vi "Main.vi"() -> ()   [LabVIEW 2021] (continued)
                    w2240 = T9 81 items=["刷新间隔", "波特率", "布尔1设置项", "布尔2设置项", "布尔3设置项", "布尔4设置项", "布尔5设置项", "布尔6设置项", "布尔7设置项", "布尔8设置项", "显控1设置", "显控2设置", "显控3设置", "显控4设置", "显控5设置", "显控6设置", "显控7设置", "显控8设置", "显控9设置", "显控10设置", "显控11设置", "显控12设置", "设控1设置", "设控2设置", "设控3设置", "设控4设置", "设控5设置", "设控6设置", "设控7设置", "设控8设置", "曲线1设置", "曲线2设置", "曲线3设置", "曲线4设置", "曲线5设置", "曲线6设置", "曲线7设置", "曲线8设置", "曲线9设置", "曲线10设置", "曲线11设置", "曲线12设置", "曲线13设置", "曲线14设置", "曲线15设置", "曲线16设置", "曲线17设置", "曲线18设置", "曲线19设置", "曲线20设置", "曲线21设置", "曲线22设置", "曲线23设置", "曲线24设置", "曲线25设置", "曲线26设置", "曲线27设置", "曲线28设置", "曲线29设置", "曲线30设置", "曲线31设置", "曲线32设置", "曲线33设置", "曲线34设置", "曲线35设置", "曲线36设置", "曲线37设置", "曲线38设置", "曲线39设置", "曲线40设置", "曲线41设置", "曲线42设置", "曲线43设置", "曲线44设置", "曲线45设置", "曲线46设置", "曲线47设置", "曲线48设置", "曲线49设置", "曲线50设置", "曲线51设置", "曲线52设置", "曲线53设置", "曲线54设置", "曲线55设置", "曲线56设置", "曲线57设置", "曲线58设置", "曲线59设置", "曲线60设置", "曲线61设置", "曲线62设置", "曲线63设置", "曲线64设置", "ID值", "数据模式"] ("DataInitDef")
                    w2244 = "曲线52" ("值")
                    n1732 = invoke on="控件配置文件" class="Tbl (严格)" method="Set Cell Value"("X Index"=1 ("X索引"), "Y Index"=w2240, "Value"="X" ("值")) -> ()  [unwired: 3 in, 6 out]
                    n1733 = invoke on="控件配置文件" class="Tbl (严格)" method="Set Cell Value"("X Index"=0 ("X索引"), "Y Index"=w2240, "Value"=w2244) -> ()  [unwired: 3 in, 6 out]
                    n1734 = property on="曲线52设置" class="Str"("Val(Sgnl)"=w2244) -> ()  [unwired: 2 in, 2 out]
                  }
                  frame "删除曲线53" {
                    w2245 = T9 82 items=["刷新间隔", "波特率", "布尔1设置项", "布尔2设置项", "布尔3设置项", "布尔4设置项", "布尔5设置项", "布尔6设置项", "布尔7设置项", "布尔8设置项", "显控1设置", "显控2设置", "显控3设置", "显控4设置", "显控5设置", "显控6设置", "显控7设置", "显控8设置", "显控9设置", "显控10设置", "显控11设置", "显控12设置", "设控1设置", "设控2设置", "设控3设置", "设控4设置", "设控5设置", "设控6设置", "设控7设置", "设控8设置", "曲线1设置", "曲线2设置", "曲线3设置", "曲线4设置", "曲线5设置", "曲线6设置", "曲线7设置", "曲线8设置", "曲线9设置", "曲线10设置", "曲线11设置", "曲线12设置", "曲线13设置", "曲线14设置", "曲线15设置", "曲线16设置", "曲线17设置", "曲线18设置", "曲线19设置", "曲线20设置", "曲线21设置", "曲线22设置", "曲线23设置", "曲线24设置", "曲线25设置", "曲线26设置", "曲线27设置", "曲线28设置", "曲线29设置", "曲线30设置", "曲线31设置", "曲线32设置", "曲线33设置", "曲线34设置", "曲线35设置", "曲线36设置", "曲线37设置", "曲线38设置", "曲线39设置", "曲线40设置", "曲线41设置", "曲线42设置", "曲线43设置", "曲线44设置", "曲线45设置", "曲线46设置", "曲线47设置", "曲线48设置", "曲线49设置", "曲线50设置", "曲线51设置", "曲线52设置", "曲线53设置", "曲线54设置", "曲线55设置", "曲线56设置", "曲线57设置", "曲线58设置", "曲线59设置", "曲线60设置", "曲线61设置", "曲线62设置", "曲线63设置", "曲线64设置", "ID值", "数据模式"] ("DataInitDef")
                    w2249 = "曲线53" ("值")
                    n1735 = invoke on="控件配置文件" class="Tbl (严格)" method="Set Cell Value"("X Index"=1 ("X索引"), "Y Index"=w2245, "Value"="X" ("值")) -> ()  [unwired: 3 in, 6 out]
                    n1736 = invoke on="控件配置文件" class="Tbl (严格)" method="Set Cell Value"("X Index"=0 ("X索引"), "Y Index"=w2245, "Value"=w2249) -> ()  [unwired: 3 in, 6 out]
                    n1737 = property on="曲线53设置" class="Str"("Val(Sgnl)"=w2249) -> ()  [unwired: 2 in, 2 out]
                  }
                  frame "删除曲线54" {
                    w2250 = T9 83 items=["刷新间隔", "波特率", "布尔1设置项", "布尔2设置项", "布尔3设置项", "布尔4设置项", "布尔5设置项", "布尔6设置项", "布尔7设置项", "布尔8设置项", "显控1设置", "显控2设置", "显控3设置", "显控4设置", "显控5设置", "显控6设置", "显控7设置", "显控8设置", "显控9设置", "显控10设置", "显控11设置", "显控12设置", "设控1设置", "设控2设置", "设控3设置", "设控4设置", "设控5设置", "设控6设置", "设控7设置", "设控8设置", "曲线1设置", "曲线2设置", "曲线3设置", "曲线4设置", "曲线5设置", "曲线6设置", "曲线7设置", "曲线8设置", "曲线9设置", "曲线10设置", "曲线11设置", "曲线12设置", "曲线13设置", "曲线14设置", "曲线15设置", "曲线16设置", "曲线17设置", "曲线18设置", "曲线19设置", "曲线20设置", "曲线21设置", "曲线22设置", "曲线23设置", "曲线24设置", "曲线25设置", "曲线26设置", "曲线27设置", "曲线28设置", "曲线29设置", "曲线30设置", "曲线31设置", "曲线32设置", "曲线33设置", "曲线34设置", "曲线35设置", "曲线36设置", "曲线37设置", "曲线38设置", "曲线39设置", "曲线40设置", "曲线41设置", "曲线42设置", "曲线43设置", "曲线44设置", "曲线45设置", "曲线46设置", "曲线47设置", "曲线48设置", "曲线49设置", "曲线50设置", "曲线51设置", "曲线52设置", "曲线53设置", "曲线54设置", "曲线55设置", "曲线56设置", "曲线57设置", "曲线58设置", "曲线59设置", "曲线60设置", "曲线61设置", "曲线62设置", "曲线63设置", "曲线64设置", "ID值", "数据模式"] ("DataInitDef")
                    w2254 = "曲线54" ("值")
                    n1738 = invoke on="控件配置文件" class="Tbl (严格)" method="Set Cell Value"("X Index"=1 ("X索引"), "Y Index"=w2250, "Value"="X" ("值")) -> ()  [unwired: 3 in, 6 out]
                    n1739 = invoke on="控件配置文件" class="Tbl (严格)" method="Set Cell Value"("X Index"=0 ("X索引"), "Y Index"=w2250, "Value"=w2254) -> ()  [unwired: 3 in, 6 out]
                    n1740 = property on="曲线54设置" class="Str"("Val(Sgnl)"=w2254) -> ()  [unwired: 2 in, 2 out]
                  }
                  frame "删除曲线55" {
                    w2255 = T9 84 items=["刷新间隔", "波特率", "布尔1设置项", "布尔2设置项", "布尔3设置项", "布尔4设置项", "布尔5设置项", "布尔6设置项", "布尔7设置项", "布尔8设置项", "显控1设置", "显控2设置", "显控3设置", "显控4设置", "显控5设置", "显控6设置", "显控7设置", "显控8设置", "显控9设置", "显控10设置", "显控11设置", "显控12设置", "设控1设置", "设控2设置", "设控3设置", "设控4设置", "设控5设置", "设控6设置", "设控7设置", "设控8设置", "曲线1设置", "曲线2设置", "曲线3设置", "曲线4设置", "曲线5设置", "曲线6设置", "曲线7设置", "曲线8设置", "曲线9设置", "曲线10设置", "曲线11设置", "曲线12设置", "曲线13设置", "曲线14设置", "曲线15设置", "曲线16设置", "曲线17设置", "曲线18设置", "曲线19设置", "曲线20设置", "曲线21设置", "曲线22设置", "曲线23设置", "曲线24设置", "曲线25设置", "曲线26设置", "曲线27设置", "曲线28设置", "曲线29设置", "曲线30设置", "曲线31设置", "曲线32设置", "曲线33设置", "曲线34设置", "曲线35设置", "曲线36设置", "曲线37设置", "曲线38设置", "曲线39设置", "曲线40设置", "曲线41设置", "曲线42设置", "曲线43设置", "曲线44设置", "曲线45设置", "曲线46设置", "曲线47设置", "曲线48设置", "曲线49设置", "曲线50设置", "曲线51设置", "曲线52设置", "曲线53设置", "曲线54设置", "曲线55设置", "曲线56设置", "曲线57设置", "曲线58设置", "曲线59设置", "曲线60设置", "曲线61设置", "曲线62设置", "曲线63设置", "曲线64设置", "ID值", "数据模式"] ("DataInitDef")
                    w2259 = "曲线55" ("值")
                    n1741 = invoke on="控件配置文件" class="Tbl (严格)" method="Set Cell Value"("X Index"=1 ("X索引"), "Y Index"=w2255, "Value"="X" ("值")) -> ()  [unwired: 3 in, 6 out]
                    n1742 = invoke on="控件配置文件" class="Tbl (严格)" method="Set Cell Value"("X Index"=0 ("X索引"), "Y Index"=w2255, "Value"=w2259) -> ()  [unwired: 3 in, 6 out]
                    n1743 = property on="曲线55设置" class="Str"("Val(Sgnl)"=w2259) -> ()  [unwired: 2 in, 2 out]
                  }
                  frame "删除曲线56" {
                    w2260 = T9 85 items=["刷新间隔", "波特率", "布尔1设置项", "布尔2设置项", "布尔3设置项", "布尔4设置项", "布尔5设置项", "布尔6设置项", "布尔7设置项", "布尔8设置项", "显控1设置", "显控2设置", "显控3设置", "显控4设置", "显控5设置", "显控6设置", "显控7设置", "显控8设置", "显控9设置", "显控10设置", "显控11设置", "显控12设置", "设控1设置", "设控2设置", "设控3设置", "设控4设置", "设控5设置", "设控6设置", "设控7设置", "设控8设置", "曲线1设置", "曲线2设置", "曲线3设置", "曲线4设置", "曲线5设置", "曲线6设置", "曲线7设置", "曲线8设置", "曲线9设置", "曲线10设置", "曲线11设置", "曲线12设置", "曲线13设置", "曲线14设置", "曲线15设置", "曲线16设置", "曲线17设置", "曲线18设置", "曲线19设置", "曲线20设置", "曲线21设置", "曲线22设置", "曲线23设置", "曲线24设置", "曲线25设置", "曲线26设置", "曲线27设置", "曲线28设置", "曲线29设置", "曲线30设置", "曲线31设置", "曲线32设置", "曲线33设置", "曲线34设置", "曲线35设置", "曲线36设置", "曲线37设置", "曲线38设置", "曲线39设置", "曲线40设置", "曲线41设置", "曲线42设置", "曲线43设置", "曲线44设置", "曲线45设置", "曲线46设置", "曲线47设置", "曲线48设置", "曲线49设置", "曲线50设置", "曲线51设置", "曲线52设置", "曲线53设置", "曲线54设置", "曲线55设置", "曲线56设置", "曲线57设置", "曲线58设置", "曲线59设置", "曲线60设置", "曲线61设置", "曲线62设置", "曲线63设置", "曲线64设置", "ID值", "数据模式"] ("DataInitDef")
                    w2264 = "曲线56" ("值")
                    n1744 = invoke on="控件配置文件" class="Tbl (严格)" method="Set Cell Value"("X Index"=1 ("X索引"), "Y Index"=w2260, "Value"="X" ("值")) -> ()  [unwired: 3 in, 6 out]
                    n1745 = invoke on="控件配置文件" class="Tbl (严格)" method="Set Cell Value"("X Index"=0 ("X索引"), "Y Index"=w2260, "Value"=w2264) -> ()  [unwired: 3 in, 6 out]
                    n1746 = property on="曲线56设置" class="Str"("Val(Sgnl)"=w2264) -> ()  [unwired: 2 in, 2 out]
                  }
                  frame "删除曲线57" {
                    w2265 = T9 86 items=["刷新间隔", "波特率", "布尔1设置项", "布尔2设置项", "布尔3设置项", "布尔4设置项", "布尔5设置项", "布尔6设置项", "布尔7设置项", "布尔8设置项", "显控1设置", "显控2设置", "显控3设置", "显控4设置", "显控5设置", "显控6设置", "显控7设置", "显控8设置", "显控9设置", "显控10设置", "显控11设置", "显控12设置", "设控1设置", "设控2设置", "设控3设置", "设控4设置", "设控5设置", "设控6设置", "设控7设置", "设控8设置", "曲线1设置", "曲线2设置", "曲线3设置", "曲线4设置", "曲线5设置", "曲线6设置", "曲线7设置", "曲线8设置", "曲线9设置", "曲线10设置", "曲线11设置", "曲线12设置", "曲线13设置", "曲线14设置", "曲线15设置", "曲线16设置", "曲线17设置", "曲线18设置", "曲线19设置", "曲线20设置", "曲线21设置", "曲线22设置", "曲线23设置", "曲线24设置", "曲线25设置", "曲线26设置", "曲线27设置", "曲线28设置", "曲线29设置", "曲线30设置", "曲线31设置", "曲线32设置", "曲线33设置", "曲线34设置", "曲线35设置", "曲线36设置", "曲线37设置", "曲线38设置", "曲线39设置", "曲线40设置", "曲线41设置", "曲线42设置", "曲线43设置", "曲线44设置", "曲线45设置", "曲线46设置", "曲线47设置", "曲线48设置", "曲线49设置", "曲线50设置", "曲线51设置", "曲线52设置", "曲线53设置", "曲线54设置", "曲线55设置", "曲线56设置", "曲线57设置", "曲线58设置", "曲线59设置", "曲线60设置", "曲线61设置", "曲线62设置", "曲线63设置", "曲线64设置", "ID值", "数据模式"] ("DataInitDef")
                    w2269 = "曲线57" ("值")
                    n1747 = invoke on="控件配置文件" class="Tbl (严格)" method="Set Cell Value"("X Index"=1 ("X索引"), "Y Index"=w2265, "Value"="X" ("值")) -> ()  [unwired: 3 in, 6 out]
                    n1748 = invoke on="控件配置文件" class="Tbl (严格)" method="Set Cell Value"("X Index"=0 ("X索引"), "Y Index"=w2265, "Value"=w2269) -> ()  [unwired: 3 in, 6 out]
                    n1749 = property on="曲线57设置" class="Str"("Val(Sgnl)"=w2269) -> ()  [unwired: 2 in, 2 out]
                  }
                  frame "删除曲线58" {
                    w2270 = T9 87 items=["刷新间隔", "波特率", "布尔1设置项", "布尔2设置项", "布尔3设置项", "布尔4设置项", "布尔5设置项", "布尔6设置项", "布尔7设置项", "布尔8设置项", "显控1设置", "显控2设置", "显控3设置", "显控4设置", "显控5设置", "显控6设置", "显控7设置", "显控8设置", "显控9设置", "显控10设置", "显控11设置", "显控12设置", "设控1设置", "设控2设置", "设控3设置", "设控4设置", "设控5设置", "设控6设置", "设控7设置", "设控8设置", "曲线1设置", "曲线2设置", "曲线3设置", "曲线4设置", "曲线5设置", "曲线6设置", "曲线7设置", "曲线8设置", "曲线9设置", "曲线10设置", "曲线11设置", "曲线12设置", "曲线13设置", "曲线14设置", "曲线15设置", "曲线16设置", "曲线17设置", "曲线18设置", "曲线19设置", "曲线20设置", "曲线21设置", "曲线22设置", "曲线23设置", "曲线24设置", "曲线25设置", "曲线26设置", "曲线27设置", "曲线28设置", "曲线29设置", "曲线30设置", "曲线31设置", "曲线32设置", "曲线33设置", "曲线34设置", "曲线35设置", "曲线36设置", "曲线37设置", "曲线38设置", "曲线39设置", "曲线40设置", "曲线41设置", "曲线42设置", "曲线43设置", "曲线44设置", "曲线45设置", "曲线46设置", "曲线47设置", "曲线48设置", "曲线49设置", "曲线50设置", "曲线51设置", "曲线52设置", "曲线53设置", "曲线54设置", "曲线55设置", "曲线56设置", "曲线57设置", "曲线58设置", "曲线59设置", "曲线60设置", "曲线61设置", "曲线62设置", "曲线63设置", "曲线64设置", "ID值", "数据模式"] ("DataInitDef")
                    w2274 = "曲线58" ("值")
                    n1750 = invoke on="控件配置文件" class="Tbl (严格)" method="Set Cell Value"("X Index"=1 ("X索引"), "Y Index"=w2270, "Value"="X" ("值")) -> ()  [unwired: 3 in, 6 out]
                    n1751 = invoke on="控件配置文件" class="Tbl (严格)" method="Set Cell Value"("X Index"=0 ("X索引"), "Y Index"=w2270, "Value"=w2274) -> ()  [unwired: 3 in, 6 out]
                    n1752 = property on="曲线58设置" class="Str"("Val(Sgnl)"=w2274) -> ()  [unwired: 2 in, 2 out]
                  }
                  frame "删除曲线59" {
                    w2275 = T9 88 items=["刷新间隔", "波特率", "布尔1设置项", "布尔2设置项", "布尔3设置项", "布尔4设置项", "布尔5设置项", "布尔6设置项", "布尔7设置项", "布尔8设置项", "显控1设置", "显控2设置", "显控3设置", "显控4设置", "显控5设置", "显控6设置", "显控7设置", "显控8设置", "显控9设置", "显控10设置", "显控11设置", "显控12设置", "设控1设置", "设控2设置", "设控3设置", "设控4设置", "设控5设置", "设控6设置", "设控7设置", "设控8设置", "曲线1设置", "曲线2设置", "曲线3设置", "曲线4设置", "曲线5设置", "曲线6设置", "曲线7设置", "曲线8设置", "曲线9设置", "曲线10设置", "曲线11设置", "曲线12设置", "曲线13设置", "曲线14设置", "曲线15设置", "曲线16设置", "曲线17设置", "曲线18设置", "曲线19设置", "曲线20设置", "曲线21设置", "曲线22设置", "曲线23设置", "曲线24设置", "曲线25设置", "曲线26设置", "曲线27设置", "曲线28设置", "曲线29设置", "曲线30设置", "曲线31设置", "曲线32设置", "曲线33设置", "曲线34设置", "曲线35设置", "曲线36设置", "曲线37设置", "曲线38设置", "曲线39设置", "曲线40设置", "曲线41设置", "曲线42设置", "曲线43设置", "曲线44设置", "曲线45设置", "曲线46设置", "曲线47设置", "曲线48设置", "曲线49设置", "曲线50设置", "曲线51设置", "曲线52设置", "曲线53设置", "曲线54设置", "曲线55设置", "曲线56设置", "曲线57设置", "曲线58设置", "曲线59设置", "曲线60设置", "曲线61设置", "曲线62设置", "曲线63设置", "曲线64设置", "ID值", "数据模式"] ("DataInitDef")
                    w2279 = "曲线59" ("值")
                    n1753 = invoke on="控件配置文件" class="Tbl (严格)" method="Set Cell Value"("X Index"=1 ("X索引"), "Y Index"=w2275, "Value"="X" ("值")) -> ()  [unwired: 3 in, 6 out]
                    n1754 = invoke on="控件配置文件" class="Tbl (严格)" method="Set Cell Value"("X Index"=0 ("X索引"), "Y Index"=w2275, "Value"=w2279) -> ()  [unwired: 3 in, 6 out]
                    n1755 = property on="曲线59设置" class="Str"("Val(Sgnl)"=w2279) -> ()  [unwired: 2 in, 2 out]
                  }
                  frame "删除曲线60" {
                    w2280 = T9 89 items=["刷新间隔", "波特率", "布尔1设置项", "布尔2设置项", "布尔3设置项", "布尔4设置项", "布尔5设置项", "布尔6设置项", "布尔7设置项", "布尔8设置项", "显控1设置", "显控2设置", "显控3设置", "显控4设置", "显控5设置", "显控6设置", "显控7设置", "显控8设置", "显控9设置", "显控10设置", "显控11设置", "显控12设置", "设控1设置", "设控2设置", "设控3设置", "设控4设置", "设控5设置", "设控6设置", "设控7设置", "设控8设置", "曲线1设置", "曲线2设置", "曲线3设置", "曲线4设置", "曲线5设置", "曲线6设置", "曲线7设置", "曲线8设置", "曲线9设置", "曲线10设置", "曲线11设置", "曲线12设置", "曲线13设置", "曲线14设置", "曲线15设置", "曲线16设置", "曲线17设置", "曲线18设置", "曲线19设置", "曲线20设置", "曲线21设置", "曲线22设置", "曲线23设置", "曲线24设置", "曲线25设置", "曲线26设置", "曲线27设置", "曲线28设置", "曲线29设置", "曲线30设置", "曲线31设置", "曲线32设置", "曲线33设置", "曲线34设置", "曲线35设置", "曲线36设置", "曲线37设置", "曲线38设置", "曲线39设置", "曲线40设置", "曲线41设置", "曲线42设置", "曲线43设置", "曲线44设置", "曲线45设置", "曲线46设置", "曲线47设置", "曲线48设置", "曲线49设置", "曲线50设置", "曲线51设置", "曲线52设置", "曲线53设置", "曲线54设置", "曲线55设置", "曲线56设置", "曲线57设置", "曲线58设置", "曲线59设置", "曲线60设置", "曲线61设置", "曲线62设置", "曲线63设置", "曲线64设置", "ID值", "数据模式"] ("DataInitDef")
                    w2284 = "曲线60" ("值")
                    n1756 = invoke on="控件配置文件" class="Tbl (严格)" method="Set Cell Value"("X Index"=1 ("X索引"), "Y Index"=w2280, "Value"="X" ("值")) -> ()  [unwired: 3 in, 6 out]
                    n1757 = invoke on="控件配置文件" class="Tbl (严格)" method="Set Cell Value"("X Index"=0 ("X索引"), "Y Index"=w2280, "Value"=w2284) -> ()  [unwired: 3 in, 6 out]
                    n1758 = property on="曲线60设置" class="Str"("Val(Sgnl)"=w2284) -> ()  [unwired: 2 in, 2 out]
                  }
                  frame "删除曲线61" {
                    w2285 = T9 90 items=["刷新间隔", "波特率", "布尔1设置项", "布尔2设置项", "布尔3设置项", "布尔4设置项", "布尔5设置项", "布尔6设置项", "布尔7设置项", "布尔8设置项", "显控1设置", "显控2设置", "显控3设置", "显控4设置", "显控5设置", "显控6设置", "显控7设置", "显控8设置", "显控9设置", "显控10设置", "显控11设置", "显控12设置", "设控1设置", "设控2设置", "设控3设置", "设控4设置", "设控5设置", "设控6设置", "设控7设置", "设控8设置", "曲线1设置", "曲线2设置", "曲线3设置", "曲线4设置", "曲线5设置", "曲线6设置", "曲线7设置", "曲线8设置", "曲线9设置", "曲线10设置", "曲线11设置", "曲线12设置", "曲线13设置", "曲线14设置", "曲线15设置", "曲线16设置", "曲线17设置", "曲线18设置", "曲线19设置", "曲线20设置", "曲线21设置", "曲线22设置", "曲线23设置", "曲线24设置", "曲线25设置", "曲线26设置", "曲线27设置", "曲线28设置", "曲线29设置", "曲线30设置", "曲线31设置", "曲线32设置", "曲线33设置", "曲线34设置", "曲线35设置", "曲线36设置", "曲线37设置", "曲线38设置", "曲线39设置", "曲线40设置", "曲线41设置", "曲线42设置", "曲线43设置", "曲线44设置", "曲线45设置", "曲线46设置", "曲线47设置", "曲线48设置", "曲线49设置", "曲线50设置", "曲线51设置", "曲线52设置", "曲线53设置", "曲线54设置", "曲线55设置", "曲线56设置", "曲线57设置", "曲线58设置", "曲线59设置", "曲线60设置", "曲线61设置", "曲线62设置", "曲线63设置", "曲线64设置", "ID值", "数据模式"] ("DataInitDef")
                    w2289 = "曲线61" ("值")
                    n1759 = invoke on="控件配置文件" class="Tbl (严格)" method="Set Cell Value"("X Index"=1 ("X索引"), "Y Index"=w2285, "Value"="X" ("值")) -> ()  [unwired: 3 in, 6 out]
                    n1760 = invoke on="控件配置文件" class="Tbl (严格)" method="Set Cell Value"("X Index"=0 ("X索引"), "Y Index"=w2285, "Value"=w2289) -> ()  [unwired: 3 in, 6 out]
                    n1761 = property on="曲线61设置" class="Str"("Val(Sgnl)"=w2289) -> ()  [unwired: 2 in, 2 out]
                  }
                  frame "删除曲线62" {
                    w2290 = T9 91 items=["刷新间隔", "波特率", "布尔1设置项", "布尔2设置项", "布尔3设置项", "布尔4设置项", "布尔5设置项", "布尔6设置项", "布尔7设置项", "布尔8设置项", "显控1设置", "显控2设置", "显控3设置", "显控4设置", "显控5设置", "显控6设置", "显控7设置", "显控8设置", "显控9设置", "显控10设置", "显控11设置", "显控12设置", "设控1设置", "设控2设置", "设控3设置", "设控4设置", "设控5设置", "设控6设置", "设控7设置", "设控8设置", "曲线1设置", "曲线2设置", "曲线3设置", "曲线4设置", "曲线5设置", "曲线6设置", "曲线7设置", "曲线8设置", "曲线9设置", "曲线10设置", "曲线11设置", "曲线12设置", "曲线13设置", "曲线14设置", "曲线15设置", "曲线16设置", "曲线17设置", "曲线18设置", "曲线19设置", "曲线20设置", "曲线21设置", "曲线22设置", "曲线23设置", "曲线24设置", "曲线25设置", "曲线26设置", "曲线27设置", "曲线28设置", "曲线29设置", "曲线30设置", "曲线31设置", "曲线32设置", "曲线33设置", "曲线34设置", "曲线35设置", "曲线36设置", "曲线37设置", "曲线38设置", "曲线39设置", "曲线40设置", "曲线41设置", "曲线42设置", "曲线43设置", "曲线44设置", "曲线45设置", "曲线46设置", "曲线47设置", "曲线48设置", "曲线49设置", "曲线50设置", "曲线51设置", "曲线52设置", "曲线53设置", "曲线54设置", "曲线55设置", "曲线56设置", "曲线57设置", "曲线58设置", "曲线59设置", "曲线60设置", "曲线61设置", "曲线62设置", "曲线63设置", "曲线64设置", "ID值", "数据模式"] ("DataInitDef")
                    w2294 = "曲线62" ("值")
                    n1762 = invoke on="控件配置文件" class="Tbl (严格)" method="Set Cell Value"("X Index"=1 ("X索引"), "Y Index"=w2290, "Value"="X" ("值")) -> ()  [unwired: 3 in, 6 out]
                    n1763 = invoke on="控件配置文件" class="Tbl (严格)" method="Set Cell Value"("X Index"=0 ("X索引"), "Y Index"=w2290, "Value"=w2294) -> ()  [unwired: 3 in, 6 out]
                    n1764 = property on="曲线62设置" class="Str"("Val(Sgnl)"=w2294) -> ()  [unwired: 2 in, 2 out]
                  }
                  frame "删除曲线63" {
                    w2295 = T9 92 items=["刷新间隔", "波特率", "布尔1设置项", "布尔2设置项", "布尔3设置项", "布尔4设置项", "布尔5设置项", "布尔6设置项", "布尔7设置项", "布尔8设置项", "显控1设置", "显控2设置", "显控3设置", "显控4设置", "显控5设置", "显控6设置", "显控7设置", "显控8设置", "显控9设置", "显控10设置", "显控11设置", "显控12设置", "设控1设置", "设控2设置", "设控3设置", "设控4设置", "设控5设置", "设控6设置", "设控7设置", "设控8设置", "曲线1设置", "曲线2设置", "曲线3设置", "曲线4设置", "曲线5设置", "曲线6设置", "曲线7设置", "曲线8设置", "曲线9设置", "曲线10设置", "曲线11设置", "曲线12设置", "曲线13设置", "曲线14设置", "曲线15设置", "曲线16设置", "曲线17设置", "曲线18设置", "曲线19设置", "曲线20设置", "曲线21设置", "曲线22设置", "曲线23设置", "曲线24设置", "曲线25设置", "曲线26设置", "曲线27设置", "曲线28设置", "曲线29设置", "曲线30设置", "曲线31设置", "曲线32设置", "曲线33设置", "曲线34设置", "曲线35设置", "曲线36设置", "曲线37设置", "曲线38设置", "曲线39设置", "曲线40设置", "曲线41设置", "曲线42设置", "曲线43设置", "曲线44设置", "曲线45设置", "曲线46设置", "曲线47设置", "曲线48设置", "曲线49设置", "曲线50设置", "曲线51设置", "曲线52设置", "曲线53设置", "曲线54设置", "曲线55设置", "曲线56设置", "曲线57设置", "曲线58设置", "曲线59设置", "曲线60设置", "曲线61设置", "曲线62设置", "曲线63设置", "曲线64设置", "ID值", "数据模式"] ("DataInitDef")
                    w2299 = "曲线63" ("值")
                    n1765 = invoke on="控件配置文件" class="Tbl (严格)" method="Set Cell Value"("X Index"=1 ("X索引"), "Y Index"=w2295, "Value"="X" ("值")) -> ()  [unwired: 3 in, 6 out]
                    n1766 = invoke on="控件配置文件" class="Tbl (严格)" method="Set Cell Value"("X Index"=0 ("X索引"), "Y Index"=w2295, "Value"=w2299) -> ()  [unwired: 3 in, 6 out]
                    n1767 = property on="曲线63设置" class="Str"("Val(Sgnl)"=w2299) -> ()  [unwired: 2 in, 2 out]
                  }
                  frame "删除曲线64" {
                    w2300 = T9 93 items=["刷新间隔", "波特率", "布尔1设置项", "布尔2设置项", "布尔3设置项", "布尔4设置项", "布尔5设置项", "布尔6设置项", "布尔7设置项", "布尔8设置项", "显控1设置", "显控2设置", "显控3设置", "显控4设置", "显控5设置", "显控6设置", "显控7设置", "显控8设置", "显控9设置", "显控10设置", "显控11设置", "显控12设置", "设控1设置", "设控2设置", "设控3设置", "设控4设置", "设控5设置", "设控6设置", "设控7设置", "设控8设置", "曲线1设置", "曲线2设置", "曲线3设置", "曲线4设置", "曲线5设置", "曲线6设置", "曲线7设置", "曲线8设置", "曲线9设置", "曲线10设置", "曲线11设置", "曲线12设置", "曲线13设置", "曲线14设置", "曲线15设置", "曲线16设置", "曲线17设置", "曲线18设置", "曲线19设置", "曲线20设置", "曲线21设置", "曲线22设置", "曲线23设置", "曲线24设置", "曲线25设置", "曲线26设置", "曲线27设置", "曲线28设置", "曲线29设置", "曲线30设置", "曲线31设置", "曲线32设置", "曲线33设置", "曲线34设置", "曲线35设置", "曲线36设置", "曲线37设置", "曲线38设置", "曲线39设置", "曲线40设置", "曲线41设置", "曲线42设置", "曲线43设置", "曲线44设置", "曲线45设置", "曲线46设置", "曲线47设置", "曲线48设置", "曲线49设置", "曲线50设置", "曲线51设置", "曲线52设置", "曲线53设置", "曲线54设置", "曲线55设置", "曲线56设置", "曲线57设置", "曲线58设置", "曲线59设置", "曲线60设置", "曲线61设置", "曲线62设置", "曲线63设置", "曲线64设置", "ID值", "数据模式"] ("DataInitDef")
                    w2304 = "曲线64" ("值")
                    n1768 = invoke on="控件配置文件" class="Tbl (严格)" method="Set Cell Value"("X Index"=1 ("X索引"), "Y Index"=w2300, "Value"="X" ("值")) -> ()  [unwired: 3 in, 6 out]
                    n1769 = invoke on="控件配置文件" class="Tbl (严格)" method="Set Cell Value"("X Index"=0 ("X索引"), "Y Index"=w2300, "Value"=w2304) -> ()  [unwired: 3 in, 6 out]
                    n1770 = property on="曲线64设置" class="Str"("Val(Sgnl)"=w2304) -> ()  [unwired: 2 in, 2 out]
                  }
                }
              }
              event "设控1": Shortcut Menu Selection (User) {
                w2307 = T9 19 items=["刷新间隔", "波特率", "布尔1设置项", "布尔2设置项", "布尔3设置项", "布尔4设置项", "布尔5设置项", "显控1设置", "显控2设置", "显控3设置", "显控4设置", "显控5设置", "显控6设置", "显控7设置", "显控8设置", "显控9设置", "显控10设置", "显控11设置", "显控12设置", "设控1设置", "设控2设置", "设控3设置", "设控4设置", "设控5设置", "设控6设置", "设控7设置", "设控8设置", "曲线1设置", "曲线2设置", "曲线3设置", "曲线4设置", "曲线5设置", "曲线6设置", "曲线7设置", "曲线8设置", "曲线9设置", "曲线10设置", "曲线11设置", "曲线12设置", "曲线13设置", "曲线14设置", "曲线15设置", "曲线16设置", "ID值"] ("DataInitDef")
                w2309 = "设控1" ("标题.文本")
                n1771 = event-data() -> ()  [unwired: 1 in, 8 out]
                n1772 = invoke on="控件配置文件" class="Tbl (严格)" method="Set Cell Value"("X Index"=1 ("X索引"), "Y Index"=w2307, "Value"="X" ("值")) -> ()  [unwired: 3 in, 6 out]
                n1773 = invoke on="控件配置文件" class="Tbl (严格)" method="Set Cell Value"("X Index"=0 ("X索引"), "Y Index"=w2307, "Value"=w2309) -> ()  [unwired: 3 in, 6 out]
                n1774 = property on="设控1" class="Str"("Caption.Text"=w2309) -> ()  [unwired: 2 in, 2 out]
                n1775 = property on="设控设置 1" class="Str"("Val(Sgnl)"=w2309) -> ()  [unwired: 2 in, 2 out]
              }
              event "设控2": Shortcut Menu Selection (User) {
                w2312 = T9 20 items=["刷新间隔", "波特率", "布尔1设置项", "布尔2设置项", "布尔3设置项", "布尔4设置项", "布尔5设置项", "显控1设置", "显控2设置", "显控3设置", "显控4设置", "显控5设置", "显控6设置", "显控7设置", "显控8设置", "显控9设置", "显控10设置", "显控11设置", "显控12设置", "设控1设置", "设控2设置", "设控3设置", "设控4设置", "设控5设置", "设控6设置", "设控7设置", "设控8设置", "曲线1设置", "曲线2设置", "曲线3设置", "曲线4设置", "曲线5设置", "曲线6设置", "曲线7设置", "曲线8设置", "曲线9设置", "曲线10设置", "曲线11设置", "曲线12设置", "曲线13设置", "曲线14设置", "曲线15设置", "曲线16设置", "ID值"] ("DataInitDef")
                w2314 = "设控2" ("标题.文本")
                n1776 = event-data() -> ()  [unwired: 1 in, 8 out]
                n1777 = invoke on="控件配置文件" class="Tbl (严格)" method="Set Cell Value"("X Index"=1 ("X索引"), "Y Index"=w2312, "Value"="X" ("值")) -> ()  [unwired: 3 in, 6 out]
                n1778 = invoke on="控件配置文件" class="Tbl (严格)" method="Set Cell Value"("X Index"=0 ("X索引"), "Y Index"=w2312, "Value"=w2314) -> ()  [unwired: 3 in, 6 out]
                n1779 = property on="设控2" class="Str"("Caption.Text"=w2314) -> ()  [unwired: 2 in, 2 out]
                n1780 = property on="设控设置 2" class="Str"("Val(Sgnl)"=w2314) -> ()  [unwired: 2 in, 2 out]
              }
              event "设控3": Shortcut Menu Selection (User) {
                w2317 = T9 21 items=["刷新间隔", "波特率", "布尔1设置项", "布尔2设置项", "布尔3设置项", "布尔4设置项", "布尔5设置项", "显控1设置", "显控2设置", "显控3设置", "显控4设置", "显控5设置", "显控6设置", "显控7设置", "显控8设置", "显控9设置", "显控10设置", "显控11设置", "显控12设置", "设控1设置", "设控2设置", "设控3设置", "设控4设置", "设控5设置", "设控6设置", "设控7设置", "设控8设置", "曲线1设置", "曲线2设置", "曲线3设置", "曲线4设置", "曲线5设置", "曲线6设置", "曲线7设置", "曲线8设置", "曲线9设置", "曲线10设置", "曲线11设置", "曲线12设置", "曲线13设置", "曲线14设置", "曲线15设置", "曲线16设置", "ID值"] ("DataInitDef")
                w2319 = "设控3" ("标题.文本")
                n1781 = event-data() -> ()  [unwired: 1 in, 8 out]
                n1782 = invoke on="控件配置文件" class="Tbl (严格)" method="Set Cell Value"("X Index"=1 ("X索引"), "Y Index"=w2317, "Value"="X" ("值")) -> ()  [unwired: 3 in, 6 out]
                n1783 = invoke on="控件配置文件" class="Tbl (严格)" method="Set Cell Value"("X Index"=0 ("X索引"), "Y Index"=w2317, "Value"=w2319) -> ()  [unwired: 3 in, 6 out]
                n1784 = property on="设控3" class="Str"("Caption.Text"=w2319) -> ()  [unwired: 2 in, 2 out]
                n1785 = property on="设控设置 3" class="Str"("Val(Sgnl)"=w2319) -> ()  [unwired: 2 in, 2 out]
              }
              event "设控4": Shortcut Menu Selection (User) {
                w2322 = T9 22 items=["刷新间隔", "波特率", "布尔1设置项", "布尔2设置项", "布尔3设置项", "布尔4设置项", "布尔5设置项", "显控1设置", "显控2设置", "显控3设置", "显控4设置", "显控5设置", "显控6设置", "显控7设置", "显控8设置", "显控9设置", "显控10设置", "显控11设置", "显控12设置", "设控1设置", "设控2设置", "设控3设置", "设控4设置", "设控5设置", "设控6设置", "设控7设置", "设控8设置", "曲线1设置", "曲线2设置", "曲线3设置", "曲线4设置", "曲线5设置", "曲线6设置", "曲线7设置", "曲线8设置", "曲线9设置", "曲线10设置", "曲线11设置", "曲线12设置", "曲线13设置", "曲线14设置", "曲线15设置", "曲线16设置", "ID值"] ("DataInitDef")
                w2324 = "设控4" ("标题.文本")
                n1786 = event-data() -> ()  [unwired: 1 in, 8 out]
                n1787 = invoke on="控件配置文件" class="Tbl (严格)" method="Set Cell Value"("X Index"=1 ("X索引"), "Y Index"=w2322, "Value"="X" ("值")) -> ()  [unwired: 3 in, 6 out]
                n1788 = invoke on="控件配置文件" class="Tbl (严格)" method="Set Cell Value"("X Index"=0 ("X索引"), "Y Index"=w2322, "Value"=w2324) -> ()  [unwired: 3 in, 6 out]
                n1789 = property on="设控4" class="Str"("Caption.Text"=w2324) -> ()  [unwired: 2 in, 2 out]
                n1790 = property on="设控设置 4" class="Str"("Val(Sgnl)"=w2324) -> ()  [unwired: 2 in, 2 out]
              }
              event "设控5": Shortcut Menu Selection (User) {
                w2329 = T9 23 items=["刷新间隔", "波特率", "布尔1设置项", "布尔2设置项", "布尔3设置项", "布尔4设置项", "布尔5设置项", "显控1设置", "显控2设置", "显控3设置", "显控4设置", "显控5设置", "显控6设置", "显控7设置", "显控8设置", "显控9设置", "显控10设置", "显控11设置", "显控12设置", "设控1设置", "设控2设置", "设控3设置", "设控4设置", "设控5设置", "设控6设置", "设控7设置", "设控8设置", "曲线1设置", "曲线2设置", "曲线3设置", "曲线4设置", "曲线5设置", "曲线6设置", "曲线7设置", "曲线8设置", "曲线9设置", "曲线10设置", "曲线11设置", "曲线12设置", "曲线13设置", "曲线14设置", "曲线15设置", "曲线16设置", "ID值"] ("DataInitDef")
                w2328 = "设控5" ("标题.文本")
                n1791 = event-data() -> ()  [unwired: 1 in, 8 out]
                n1792 = invoke on="控件配置文件" class="Tbl (严格)" method="Set Cell Value"("X Index"=1 ("X索引"), "Y Index"=w2329, "Value"="X" ("值")) -> ()  [unwired: 3 in, 6 out]
                n1793 = invoke on="控件配置文件" class="Tbl (严格)" method="Set Cell Value"("X Index"=0 ("X索引"), "Y Index"=w2329, "Value"=w2328) -> ()  [unwired: 3 in, 6 out]
                n1794 = property on="设控5" class="Str"("Caption.Text"=w2328) -> ()  [unwired: 2 in, 2 out]
                n1795 = property on="设控设置 5" class="Str"("Val(Sgnl)"=w2328) -> ()  [unwired: 2 in, 2 out]
              }
              event "设控6": Shortcut Menu Selection (User) {
                w2334 = T9 24 items=["刷新间隔", "波特率", "布尔1设置项", "布尔2设置项", "布尔3设置项", "布尔4设置项", "布尔5设置项", "显控1设置", "显控2设置", "显控3设置", "显控4设置", "显控5设置", "显控6设置", "显控7设置", "显控8设置", "显控9设置", "显控10设置", "显控11设置", "显控12设置", "设控1设置", "设控2设置", "设控3设置", "设控4设置", "设控5设置", "设控6设置", "设控7设置", "设控8设置", "曲线1设置", "曲线2设置", "曲线3设置", "曲线4设置", "曲线5设置", "曲线6设置", "曲线7设置", "曲线8设置", "曲线9设置", "曲线10设置", "曲线11设置", "曲线12设置", "曲线13设置", "曲线14设置", "曲线15设置", "曲线16设置", "ID值"] ("DataInitDef")
                w2333 = "设控6" ("标题.文本")
                n1796 = event-data() -> ()  [unwired: 1 in, 8 out]
                n1797 = invoke on="控件配置文件" class="Tbl (严格)" method="Set Cell Value"("X Index"=1 ("X索引"), "Y Index"=w2334, "Value"="X" ("值")) -> ()  [unwired: 3 in, 6 out]
                n1798 = invoke on="控件配置文件" class="Tbl (严格)" method="Set Cell Value"("X Index"=0 ("X索引"), "Y Index"=w2334, "Value"=w2333) -> ()  [unwired: 3 in, 6 out]
                n1799 = property on="设控6" class="Str"("Caption.Text"=w2333) -> ()  [unwired: 2 in, 2 out]
                n1800 = property on="设控设置 6" class="Str"("Val(Sgnl)"=w2333) -> ()  [unwired: 2 in, 2 out]
              }
              event "设控7": Shortcut Menu Selection (User) {
                w2337 = T9 25 items=["刷新间隔", "波特率", "布尔1设置项", "布尔2设置项", "布尔3设置项", "布尔4设置项", "布尔5设置项", "显控1设置", "显控2设置", "显控3设置", "显控4设置", "显控5设置", "显控6设置", "显控7设置", "显控8设置", "显控9设置", "显控10设置", "显控11设置", "显控12设置", "设控1设置", "设控2设置", "设控3设置", "设控4设置", "设控5设置", "设控6设置", "设控7设置", "设控8设置", "曲线1设置", "曲线2设置", "曲线3设置", "曲线4设置", "曲线5设置", "曲线6设置", "曲线7设置", "曲线8设置", "曲线9设置", "曲线10设置", "曲线11设置", "曲线12设置", "曲线13设置", "曲线14设置", "曲线15设置", "曲线16设置", "ID值"] ("DataInitDef")
                w2339 = "设控7" ("标题.文本")
                n1801 = event-data() -> ()  [unwired: 1 in, 8 out]
                n1802 = invoke on="控件配置文件" class="Tbl (严格)" method="Set Cell Value"("X Index"=1 ("X索引"), "Y Index"=w2337, "Value"="X" ("值")) -> ()  [unwired: 3 in, 6 out]
                n1803 = invoke on="控件配置文件" class="Tbl (严格)" method="Set Cell Value"("X Index"=0 ("X索引"), "Y Index"=w2337, "Value"=w2339) -> ()  [unwired: 3 in, 6 out]
                n1804 = property on="设控7" class="Str"("Caption.Text"=w2339) -> ()  [unwired: 2 in, 2 out]
                n1805 = property on="设控设置 7" class="Str"("Val(Sgnl)"=w2339) -> ()  [unwired: 2 in, 2 out]
              }
              event "设控8": Shortcut Menu Selection (User) {
                w2342 = T9 26 items=["刷新间隔", "波特率", "布尔1设置项", "布尔2设置项", "布尔3设置项", "布尔4设置项", "布尔5设置项", "显控1设置", "显控2设置", "显控3设置", "显控4设置", "显控5设置", "显控6设置", "显控7设置", "显控8设置", "显控9设置", "显控10设置", "显控11设置", "显控12设置", "设控1设置", "设控2设置", "设控3设置", "设控4设置", "设控5设置", "设控6设置", "设控7设置", "设控8设置", "曲线1设置", "曲线2设置", "曲线3设置", "曲线4设置", "曲线5设置", "曲线6设置", "曲线7设置", "曲线8设置", "曲线9设置", "曲线10设置", "曲线11设置", "曲线12设置", "曲线13设置", "曲线14设置", "曲线15设置", "曲线16设置", "ID值"] ("DataInitDef")
                w2344 = "设控8" ("标题.文本")
                n1806 = event-data() -> ()  [unwired: 1 in, 8 out]
                n1807 = invoke on="控件配置文件" class="Tbl (严格)" method="Set Cell Value"("X Index"=1 ("X索引"), "Y Index"=w2342, "Value"="X" ("值")) -> ()  [unwired: 3 in, 6 out]
                n1808 = invoke on="控件配置文件" class="Tbl (严格)" method="Set Cell Value"("X Index"=0 ("X索引"), "Y Index"=w2342, "Value"=w2344) -> ()  [unwired: 3 in, 6 out]
                n1809 = property on="设控8" class="Str"("Caption.Text"=w2344) -> ()  [unwired: 2 in, 2 out]
                n1810 = property on="设控设置 8" class="Str"("Val(Sgnl)"=w2344) -> ()  [unwired: 2 in, 2 out]
              }
            }
          }
          frame #4 {
            # "导入表格参数处理代码"
            n1811 = event shown="[1] \"选择参数表\": 值改变" {
              selector: _ -> [_ _]
              dyn-events: _ -> [_ _]
              timeout: 0 -> [_ _]
              event Timeout {
                n1812 = event-data() -> ()  [unwired: 1 in, 3 out]
              }
              event "选择参数表": Value Change {
                # "读取指定的EXCEL文件，从中导入要显示的参数"
                n1813 = event-data() -> ()  [unwired: 1 in, 3 out]
                n1814 = flat-sequence {
                  tunnel: ["选择参数表"] -> w2351
                  tunnel: [w2354] -> w2350
                  tunnel: [w2353] -> w2349
                  tunnel: w2351 -> [w2366]
                  tunnel: w2350 -> [w2365]
                  tunnel: w2349 -> [w2361]
                  tunnel: [w2366] -> w2348
                  tunnel: [w2365] -> w2347
                  tunnel: [w2360] -> w2346
                  tunnel: w2348 -> [w2377]
                  tunnel: w2347 -> [w2378]
                  tunnel: w2346 -> [w2376]
                  frame #0 {
                    n1815 = call <vilib>:"Create Report.vi"("report type"=Report_Type."Excel", "template (empty)"="选择参数表") -> ("report out"=w2358:refnum<class "NI_report.lvclass">, "error out"=w2357:errorcluster)  [unwired: 12 in]
                    n1816 = call <vilib>:"Excel Get Last Row.vi"("report in"=w2358, "error in (no error)"=w2357) -> ("report out"=w2356:refnum<class "NI_report.lvclass">, "MS Office parameters out"=w2353:T11, "error out"=w2355:errorcluster)  [unwired: 11 in]
                    n1817 = call-dynamic "Dispose Report.vi"("report in"=w2356, "error in (no error)"=w2355) -> ("error out"=w2354:errorcluster)  [unwired: 13 in]
                  }
                  frame #1 {
                    n1818 = Unbundle By Name(w2361) -> ("position (excel)"=w2362:cluster{"row":i32, "column":i32})
                    n1819 = Unbundle By Name(w2362) -> ("row"=w2363:i32)
                    n1820 = Bundle By Name(cluster=w2362, "row"=w2363, "column"=9) -> (w2360:cluster{"row":i32, "column":i32})
                  }
                  frame #2 {
                    n1821 = call "Excel Read.vi"("error in (no error)"=w2378, "end (-1, -1)"=w2376, "start (-1, -1)"=cluster{"row":i32, "column":i32} {"row"=0, "column"=0}, "template (empty)"=w2377) -> ("error out"=w2375:errorcluster, "Array"=w2370:string[][])  [unwired: 6 in]
                    n1822 = Unbundle By Name(w2375) -> ("status"=w2373:bool, "source"=w2374:string)  [unwired: 1 out]
                    n1823 = Array To Spreadsheet String(array=w2370, 3:"%s" ("格式字符串")) -> (spreadsheet string=w2372:string)  [unwired: 1 in]
                    n1824 = call <vilib>:"Application Directory.vi"() -> ("Application Directory"=w2368:path)
                    n1825 = call "显示对话框信息"("Enable"=w2373, "Message"=w2374) -> ()  [unwired: 8 in, 2 out]
                    n1826 = Build Path(base path=w2368, name or relative path="Config\\DATA.txt" ("名称或相对路径")) -> (appended path=w2367:path)
                    n1827 = Write to Text File(file (use dialog)=w2367, text=w2372) -> ()  [unwired: 2 in, 3 out]
                  }
                }
              }
            }
          }
        }
      }
      frame #2 {
        # "更新与显示有关的控件"
        n1828 = Quotient & Remainder(x="i2", y=10) -> (x-y*floor(x/y)=w2383:u32)  [unwired: 1 out]
        n1829 = Increment(x="i2") -> (x+1=w2382:u32)
        n1830 = Equal To 0?(x=w2383) -> (x = 0?=w2380:bool)
        n1831 = local write "i2"(w2382) -> ()
        n1832 = case shown="真" w2380 {
          frame False {
          }
          frame True {
            n1833 = stacked-sequence {
              frame #0 {
                # "发送跟新的值"
                n1834 = property on="CANBURF" class="Arr (严格)"() -> ("Value"=w2390:u32[][])  [unwired: 2 in, 2 out]
                n1835 = event shown="[1] \"要发送的数据\": 值改变" {
                  selector: _ -> [_ _]
                  dyn-events: _ -> [_ _]
                  timeout: 0 -> [_ _]
                  tunnel: w2390 -> [w2392 w2397]
                  tunnel: [w2392 w2398] -> w2388
                  event Timeout {
                    n1836 = event-data() -> ()  [unwired: 1 in, 3 out]
                  }
                  event "要发送的数据": Value Change {
                    # "实时修改参数设置控件更新的值"
                    n1837 = event-data() -> ("NewVal"=w2399:cluster{"地址":u16, "数据":i32, "行数":i32, "ID":i32})  [unwired: 1 in, 5 out]
                    n1838 = Unbundle(w2399) -> ("地址"=w2393:u16, "数据"=w2394:i32)  [unwired: 2 out]
                    n1839 = flat-sequence {
                      tunnel: w2394 -> [w2404]
                      tunnel: w2397 -> [w2401]
                      tunnel: [w2404] -> w2396
                      tunnel: [w2402] -> w2395
                      tunnel: w2393 -> [w2403]
                      tunnel: w2396 -> [w2420]
                      tunnel: w2395 -> [w2419]
                      tunnel: [w2417] -> w2398
                      tunnel: w2397 -> [w2416]
                      frame #0 {
                        n1840 = local read "当前显示表格总行数"() -> (w2400:i32)
                        n1841 = while {
                          tunnel: [w2409] -> w2402
                          tunnel: w2401 -> [w2408]
                          tunnel: w2403 -> [w2406]
                          tunnel: w2400 -> [w2405]
                          i -> [w2411]
                          stop <- w2413 stop-if-true
                          # "查找CANBURF中与表格第0行相匹配的行数"
                          n1842 = Greater?(x=w2411, y=w2405) -> (0:w2414:bool)
                          n1843 = Index Array(array=w2408, index (row)=w2411, index (col)=0 ("禁用的索引 (列)")) -> (element=w2407:u32)
                          n1844 = Equal?(x=w2407, y=w2406) -> (x = y?=w2412:bool)
                          n1845 = Or(x=w2412, y=w2414) -> (x .or. y?=w2413:bool)
                          n1846 = Select(t=w2411, s=w2412, f=0) -> (s? t:f=w2409:i32)
                        }
                      }
                      frame #1 {
                        n1847 = Replace Array Subset(array=w2416, new element=w2420, index (row)=w2419, index (col)=1 ("禁用的索引 (列)")) -> (w2417:u32[][])
                        n1848 = local write "CANBURF"(w2417) -> ()
                      }
                    }
                  }
                }
                n1849 = local read "表格"() -> (w2387:string[][])
                n1850 = local read "当前显示表格总行数"() -> (w2389:i32)
                n1851 = call "表格显示内容刷新V2.vi"("数据模式"="数据模式", "表格"=w2387, "CANBURF"=w2388, "当前显示表格总行数"=w2389) -> ("输出数组"=w2386:string[][])  [unwired: 7 in]
                n1852 = property on="表格" class="Tbl (严格)"("Value"=w2386) -> ()  [unwired: 2 in, 2 out]
              }
              frame #1 {
                # "故障状态显示，请修改config文件夹下的ERROR.TXT故障字典的内容，务必填写正确的故障地址"
                n1853 = stacked-sequence {
                  frame #0 {
                    # "从故障字典中获取代表故障信息的地址"
                    n1854 = local read "故障地址"() -> (w2424:string[])
                    n1855 = local read "故障字典"() -> (w2421:string[][])
                    n1856 = Array Size(array=w2424) -> (size(s)=w2425:i32)
                    n1857 = Delete From Array "删除数组元素"(array=w2424, length=w2425) -> (array with subset deleted=w2423:string[])  [unwired: 1 in, 1 out]
                    n1858 = for "For循环" {
                      tunnel: w2421 -> [w2430] mode=indexing
                      shift-right: [w2429] -> w2422
                      shift-left: w2423 -> [w2428]
                      n1859 = Index Array(array=w2430, index=1 ("禁用的索引 (列)")) -> (element=w2431:string)
                      n1860 = Index Array(array=w2430, index=0 ("禁用的索引 (列)")) -> (element=w2434:string)
                      n1861 = Equal?(x=w2434, y="") -> ()  [unwired: 1 out]
                      n1862 = Equal?(x=w2434, y="地址") -> (x = y?=w2432:bool)
                      n1863 = case shown="真" w2432 {
                        tunnel: w2431 -> [_ w2439]
                        tunnel: [w2436 w2438] -> w2429
                        tunnel: w2428 -> [w2436 w2437]
                        frame False {
                        }
                        frame True {
                          n1864 = Build Array (concatenate)(w2437, w2439) -> (w2438:string[])
                        }
                      }
                    }
                    "故障地址" <- w2422
                  }
                  frame #1 {
                    # "通过故障地址搜索表格的对应位置获取故障信息"
                    n1865 = local read "故障地址"() -> (w2442:string[])
                    n1866 = local read "表格"() -> (w2441:string[][])
                    n1867 = for "For循环" {
                      tunnel: w2442 -> [w2443] mode=indexing
                      tunnel: w2441 -> [w2445]
                      tunnel: [w2444] -> w2440 mode=indexing
                      n1868 = while {
                        tunnel: w2445 -> [w2449]
                        tunnel: w2443 -> [w2454]
                        tunnel: [w2447] -> w2444
                        i -> [w2448]
                        stop <- w2451 stop-if-true
                        n1869 = Index Array(array=w2449, index (row)=w2448, index (col)=1 ("禁用的索引 (列)")) -> (element=w2446:string)
                        n1870 = Equal?(x=w2446, y="") -> (x = y?=w2452:bool)
                        n1871 = Equal?(x=w2454, y=w2446) -> (x = y?=w2450:bool)
                        n1872 = Or(x=w2450, y=w2452) -> (x .or. y?=w2451:bool)
                        n1873 = case shown="真" w2450 {
                          tunnel: w2449 -> [_ w2459]
                          tunnel: w2448 -> [_ w2458]
                          tunnel: [_ w2456] -> w2447
                          frame False {
                          }
                          frame True {
                            n1874 = Index Array(array=w2459, index (row)=w2458, index (col)=2 ("禁用的索引 (列)")) -> (element=w2456:string)
                          }
                        }
                      }
                    }
                    "故障信息" <- w2440
                  }
                  frame #2 {
                    # "将故障信息中的每一个位于故障字典的内容对应起来，并将等于1的故障位的内容挑选出来"
                    n1875 = local read "故障信息"() -> (w2464:string[])
                    n1876 = local read "故障内容"() -> (w2463:string[])
                    n1877 = local read "故障字典"() -> (w2462:string[][])
                    n1878 = local read "数据模式"() -> (w2460:bool)
                    n1879 = call "故障处理.vi"("数据模式"=w2460, "故障字典"=w2462, "原故障内容"=w2463, "故障信息"=w2464) -> ("故障内容"=w2461:string[])  [unwired: 7 in]
                    n1880 = local write "故障内容"(w2461) -> ()
                  }
                  frame #3 {
                    # "将对应故障内容显示在屏幕上"
                    n1881 = local read "故障内容"() -> (w2470:string[])
                    n1882 = Array To Spreadsheet String(delimiter (Tab)="\n" ("分隔符(Tab)"), array=w2470, 3:"%s" ("格式字符串")) -> (spreadsheet string=w2465:string)
                    n1883 = Not Equal?(x=w2465, y="") -> (x != y?=w2466:bool)
                    n1884 = case shown="真" w2466 {
                      tunnel: w2465 -> [_ w2474]
                      frame False {
                        n1885 = property on="状态显示" class="Str"("Text.TextColor"=u32 0 ("文本.文本颜色:文本颜色")) -> ()  [unwired: 2 in, 2 out]
                        n1886 = local write "状态显示"("无故障" ("状态显示")) -> ()
                      }
                      frame True {
                        n1887 = local write "状态显示"(w2474) -> ()
                        n1888 = property on="状态显示" class="Str"("Text.TextColor"=u32 16711680 ("文本.文本颜色:文本颜色")) -> ()  [unwired: 2 in, 2 out]
                      }
                    }
                  }
                }
              }
              frame #2 {
                w2487 = T9 21 items=["刷新间隔", "波特率", "布尔1设置项", "布尔2设置项", "布尔3设置项", "布尔4设置项", "布尔5设置项", "显控1设置", "显控2设置", "显控3设置", "显控4设置", "显控5设置", "显控6设置", "显控7设置", "显控8设置", "显控9设置", "显控10设置", "显控11设置", "显控12设置", "设控1设置", "设控2设置", "设控3设置", "设控4设置", "设控5设置", "设控6设置", "设控7设置", "设控8设置", "曲线1设置", "曲线2设置", "曲线3设置", "曲线4设置", "曲线5设置", "曲线6设置", "曲线7设置", "曲线8设置", "曲线9设置", "曲线10设置", "曲线11设置", "曲线12设置", "曲线13设置", "曲线14设置", "曲线15设置", "曲线16设置", "ID值"] ("DataInitDef")
                w2488 = T9 20 items=["刷新间隔", "波特率", "布尔1设置项", "布尔2设置项", "布尔3设置项", "布尔4设置项", "布尔5设置项", "显控1设置", "显控2设置", "显控3设置", "显控4设置", "显控5设置", "显控6设置", "显控7设置", "显控8设置", "显控9设置", "显控10设置", "显控11设置", "显控12设置", "设控1设置", "设控2设置", "设控3设置", "设控4设置", "设控5设置", "设控6设置", "设控7设置", "设控8设置", "曲线1设置", "曲线2设置", "曲线3设置", "曲线4设置", "曲线5设置", "曲线6设置", "曲线7设置", "曲线8设置", "曲线9设置", "曲线10设置", "曲线11设置", "曲线12设置", "曲线13设置", "曲线14设置", "曲线15设置", "曲线16设置", "ID值"] ("DataInitDef")
                w2489 = T9 22 items=["刷新间隔", "波特率", "布尔1设置项", "布尔2设置项", "布尔3设置项", "布尔4设置项", "布尔5设置项", "显控1设置", "显控2设置", "显控3设置", "显控4设置", "显控5设置", "显控6设置", "显控7设置", "显控8设置", "显控9设置", "显控10设置", "显控11设置", "显控12设置", "设控1设置", "设控2设置", "设控3设置", "设控4设置", "设控5设置", "设控6设置", "设控7设置", "设控8设置", "曲线1设置", "曲线2设置", "曲线3设置", "曲线4设置", "曲线5设置", "曲线6设置", "曲线7设置", "曲线8设置", "曲线9设置", "曲线10设置", "曲线11设置", "曲线12设置", "曲线13设置", "曲线14设置", "曲线15设置", "曲线16设置", "ID值"] ("DataInitDef")
                w2490 = T9 23 items=["刷新间隔", "波特率", "布尔1设置项", "布尔2设置项", "布尔3设置项", "布尔4设置项", "布尔5设置项", "显控1设置", "显控2设置", "显控3设置", "显控4设置", "显控5设置", "显控6设置", "显控7设置", "显控8设置", "显控9设置", "显控10设置", "显控11设置", "显控12设置", "设控1设置", "设控2设置", "设控3设置", "设控4设置", "设控5设置", "设控6设置", "设控7设置", "设控8设置", "曲线1设置", "曲线2设置", "曲线3设置", "曲线4设置", "曲线5设置", "曲线6设置", "曲线7设置", "曲线8设置", "曲线9设置", "曲线10设置", "曲线11设置", "曲线12设置", "曲线13设置", "曲线14设置", "曲线15设置", "曲线16设置", "ID值"] ("DataInitDef")
                w2491 = T9 24 items=["刷新间隔", "波特率", "布尔1设置项", "布尔2设置项", "布尔3设置项", "布尔4设置项", "布尔5设置项", "显控1设置", "显控2设置", "显控3设置", "显控4设置", "显控5设置", "显控6设置", "显控7设置", "显控8设置", "显控9设置", "显控10设置", "显控11设置", "显控12设置", "设控1设置", "设控2设置", "设控3设置", "设控4设置", "设控5设置", "设控6设置", "设控7设置", "设控8设置", "曲线1设置", "曲线2设置", "曲线3设置", "曲线4设置", "曲线5设置", "曲线6设置", "曲线7设置", "曲线8设置", "曲线9设置", "曲线10设置", "曲线11设置", "曲线12设置", "曲线13设置", "曲线14设置", "曲线15设置", "曲线16设置", "ID值"] ("DataInitDef")
                w2492 = T9 25 items=["刷新间隔", "波特率", "布尔1设置项", "布尔2设置项", "布尔3设置项", "布尔4设置项", "布尔5设置项", "显控1设置", "显控2设置", "显控3设置", "显控4设置", "显控5设置", "显控6设置", "显控7设置", "显控8设置", "显控9设置", "显控10设置", "显控11设置", "显控12设置", "设控1设置", "设控2设置", "设控3设置", "设控4设置", "设控5设置", "设控6设置", "设控7设置", "设控8设置", "曲线1设置", "曲线2设置", "曲线3设置", "曲线4设置", "曲线5设置", "曲线6设置", "曲线7设置", "曲线8设置", "曲线9设置", "曲线10设置", "曲线11设置", "曲线12设置", "曲线13设置", "曲线14设置", "曲线15设置", "曲线16设置", "ID值"] ("DataInitDef")
                w2485 = T9 19 items=["刷新间隔", "波特率", "布尔1设置项", "布尔2设置项", "布尔3设置项", "布尔4设置项", "布尔5设置项", "显控1设置", "显控2设置", "显控3设置", "显控4设置", "显控5设置", "显控6设置", "显控7设置", "显控8设置", "显控9设置", "显控10设置", "显控11设置", "显控12设置", "设控1设置", "设控2设置", "设控3设置", "设控4设置", "设控5设置", "设控6设置", "设控7设置", "设控8设置", "曲线1设置", "曲线2设置", "曲线3设置", "曲线4设置", "曲线5设置", "曲线6设置", "曲线7设置", "曲线8设置", "曲线9设置", "曲线10设置", "曲线11设置", "曲线12设置", "曲线13设置", "曲线14设置", "曲线15设置", "曲线16设置", "ID值"] ("DataInitDef")
                w2486 = T9 26 items=["刷新间隔", "波特率", "布尔1设置项", "布尔2设置项", "布尔3设置项", "布尔4设置项", "布尔5设置项", "显控1设置", "显控2设置", "显控3设置", "显控4设置", "显控5设置", "显控6设置", "显控7设置", "显控8设置", "显控9设置", "显控10设置", "显控11设置", "显控12设置", "设控1设置", "设控2设置", "设控3设置", "设控4设置", "设控5设置", "设控6设置", "设控7设置", "设控8设置", "曲线1设置", "曲线2设置", "曲线3设置", "曲线4设置", "曲线5设置", "曲线6设置", "曲线7设置", "曲线8设置", "曲线9设置", "曲线10设置", "曲线11设置", "曲线12设置", "曲线13设置", "曲线14设置", "曲线15设置", "曲线16设置", "ID值"] ("DataInitDef")
                w2498 = T9 8 items=["刷新间隔", "波特率", "布尔1设置项", "布尔2设置项", "布尔3设置项", "布尔4设置项", "布尔5设置项", "显控1设置", "显控2设置", "显控3设置", "显控4设置", "显控5设置", "显控6设置", "显控7设置", "显控8设置", "显控9设置", "显控10设置", "显控11设置", "显控12设置", "设控1设置", "设控2设置", "设控3设置", "设控4设置", "设控5设置", "设控6设置", "设控7设置", "设控8设置", "曲线1设置", "曲线2设置", "曲线3设置", "曲线4设置", "曲线5设置", "曲线6设置", "曲线7设置", "曲线8设置", "曲线9设置", "曲线10设置", "曲线11设置", "曲线12设置", "曲线13设置", "曲线14设置", "曲线15设置", "曲线16设置", "ID值"] ("DataInitDef")
